vi "exec.vi"(8 "error in (no error)":errorcluster, 10 "context":refnum<class "IContextThisComponent.lvclass">, 11 "Disable in":refnum<class "Disable.lvclass">) -> (0 "error out":errorcluster, 2 "context 2":refnum<class "IContextThisComponent.lvclass">, 3 "Disable out":refnum<class "Disable.lvclass">)   [LabVIEW 2012, in "Commands.lvlib" / "Disable.lvclass"]
uses:
  Disable.lvclass
  IContextThisComponent/IContextThisComponent.lvclass
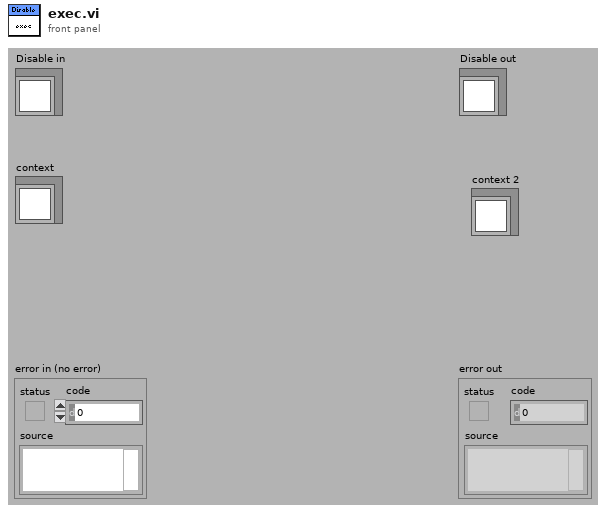
[diagram p1: front panel]
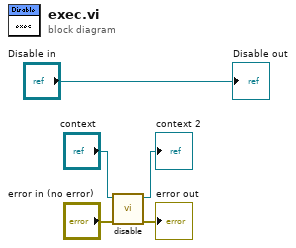
[diagram p0: block diagram]
diagram:
  n1 = call-dynamic "disable.vi"("error in (no error)"="error in (no error)", "IContextThisComponent in"="context") -> ("error out"=→"error out":errorcluster, "IContextThisComponent out"=→"context 2":refnum<class "IContextThisComponent.lvclass">)  [unwired: 8 in]
  "Disable out" <- "Disable in"
